vi "DiffVIs.vi"(6 "Title Prefix In":string, 8 "error in":errorcluster, 9 "Picture Save Location":path, 10 "VI Path 2":path, 11 "VI Path 1":path) -> (0 "error out":errorcluster, 2 "diff file":path)   [LabVIEW 2015]
uses:
  Utilities/Arguments.ctl
  Screenshots/VI Screenshots.ctl
  Screenshots/Screenshot Info.ctl
  Screenshots/Screenshot Type.ctl
  Utilities/FilePaths.ctl
  Utilities/VIDiff_Utilities.lvlib
  Screenshots/VIDiff_Screenshots.lvlib
panel:
  out "Description":string
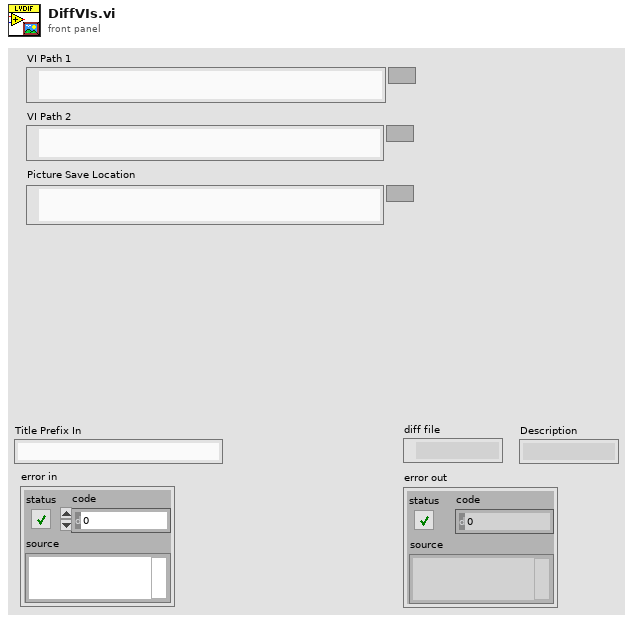
[diagram p1: front panel]
types:
  T1 = typedef "VIDiff_Screenshots.lvlib/Screenshot Type.ctl" = enum16{"Unknown", "Front Panel", "Connector Pane", "Block Diagram", "VI Hierarchy"}
  T2 = typedef "VIDiff_Screenshots.lvlib/VI Screenshots.ctl" = cluster{"Front Panel Screenshots":T3[], "Block Diagram Screenshots":T3[], "Connector Pane Screenshots":T3[], "VI Hierarchy Screenshots":T3[], "Unknown Screenshots":T3[], "vi reference":refnum<vi>, "File Paths":cluster{"File Path":path, "Container Path":path}}
  T3 = typedef "VIDiff_Screenshots.lvlib/Screenshot Info.ctl" = cluster{"Screenshot Path":path, "Screenshot Type":T1, "VI Paths":T4}
  T4 = typedef "VIDiff_Utilities.lvlib/FilePaths.ctl" = cluster{"File Path":path, "Container Path":path}
  T5 = typedef "VIDiff_Utilities.lvlib/Arguments.ctl" = cluster{"VI 1 Path":path, "VI 2 Path":path, "Picture Save Location":path, "Screenshot Title":string}
  T6 = typedef "VIDiff_Utilities.lvlib/Output Folders.ctl" = cluster{"combined":path, "vi1shots":path, "vi2shots":path, "Picture Save Location":path}
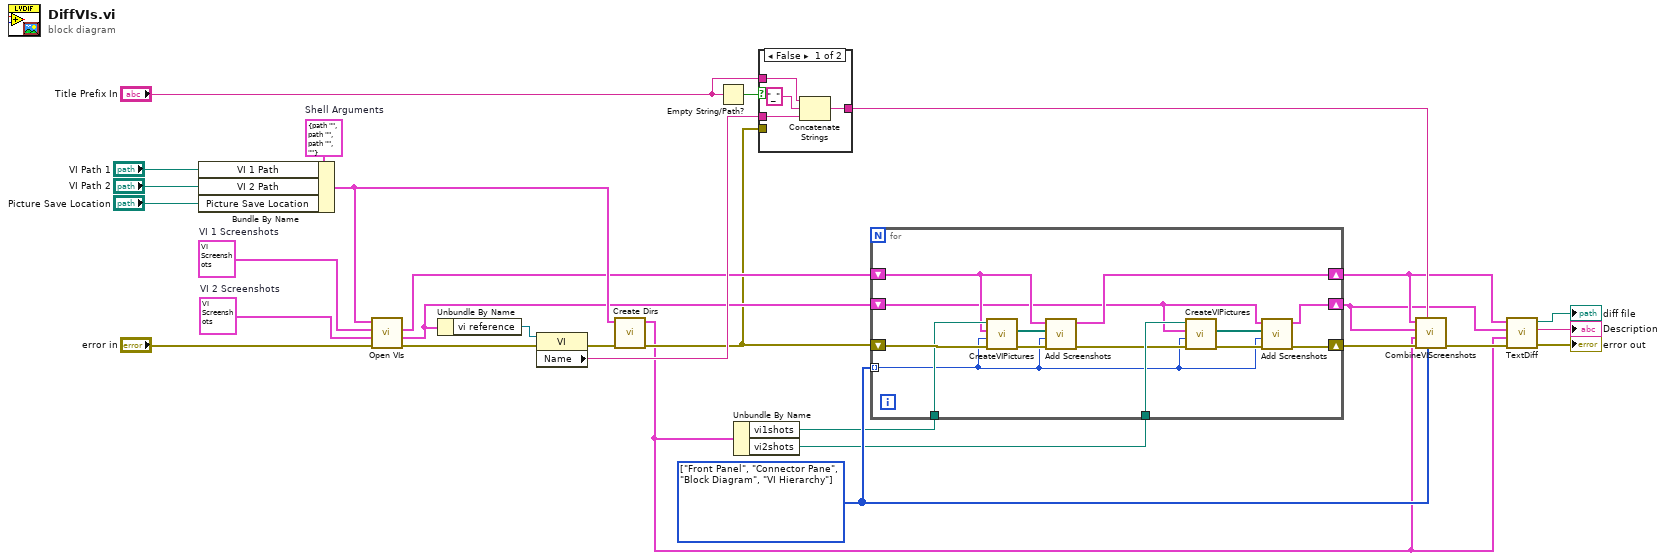
[diagram p0: block diagram]
diagram:
  w17 = T1[] [enum."Front Panel", enum."Connector Pane", enum."Block Diagram", enum."VI Hierarchy"] items=["Unknown", "Front Panel", "Connector Pane", "Block Diagram", "VI Hierarchy"]
  w6 = T2 {"Front Panel Screenshots"=[], "Block Diagram Screenshots"=[], "Connector Pane Screenshots"=[], "VI Hierarchy Screenshots"=[], "Unknown Screenshots"=[], "vi reference"=refnum, "File Paths"={"File Path"=path "", "Container Path"=path ""}}  # VI 2 Screenshots
  w20 = T2 {"Front Panel Screenshots"=[], "Block Diagram Screenshots"=[], "Connector Pane Screenshots"=[], "VI Hierarchy Screenshots"=[], "Unknown Screenshots"=[], "vi reference"=refnum, "File Paths"={"File Path"=path "", "Container Path"=path ""}}  # VI 1 Screenshots
  w29 = T5 {"VI 1 Path"=path "", "VI 2 Path"=path "", "Picture Save Location"=path "", "Screenshot Title"=""}  # Shell Arguments
  n1 = Bundle By Name(cluster=w29, "VI 1 Path"="VI Path 1", "VI 2 Path"="VI Path 2", "Picture Save Location"="Picture Save Location") -> (w21:T5)
  n2 = call "Open VIs.vi"("error in (no error)"="error in", "VI 2 Screenshots 2"=w6, "VI 1 Screenshots"=w20, "Shell Arguments"=w21) -> ("error out"=w10:errorcluster, "VI 2 Screenshots out"=w7:T2, "VI 1 Screenshots out"=w8:T2)  [unwired: 5 in]
  n3 = Unbundle By Name(w7) -> ("vi reference"=w22:refnum<vi>)
  n4 = property class="VI"(reference=w22, error in=w10) -> (error out=w9:errorcluster, "Name"=w13:string)  [unwired: 1 out]
  n5 = call "Create Dirs.vi"("error in (no error)"=w9, "Shell Arguments"=w21) -> ("error out"=w5:errorcluster, "Output Folders"=w2:T6)  [unwired: 8 in]
  n6 = Empty String/Path?(string/path="Title Prefix In") -> (empty?=w19:bool)
  n7 = Unbundle By Name(w2) -> ("vi1shots"=w16:path, "vi2shots"=w15:path)
  n8 = case shown="False" w19 {
    tunnel: w13 -> [w33 w34]
    tunnel: [w32 w34] -> w23
    tunnel: "Title Prefix In" -> [w30 _]
    tunnel: w5 -> [_ _]
    frame False {
      n9 = Concatenate Strings(w30, "_" ("string"), w33) -> (w32:string)
    }
    frame True {
    }
  }
  n10 = for {
    tunnel: w17 -> [w35] mode=indexing
    shift-right: [w43] -> w18
    shift-left: w5 -> [w48]
    tunnel: w16 -> [w47]
    tunnel: w15 -> [w46]
    shift-right: [w42] -> w4
    shift-left: w8 -> [w40]
    shift-right: [w41] -> w3
    shift-left: w7 -> [w39]
    n11 = call "CreateVIPictures.vi"("error in (no error)"=w48, "Capture Target"=w35, "VI 1 Screenshots"=w40, "Picture Save Location"=w47) -> ("error out"=w38:errorcluster, "Screenshot Files"=w45:path[])  [unwired: 6 in]
    n12 = call "Add Screenshots.vi"("error in (no error)"=w38, "Screenshot Type"=w35, "Screenshot Paths"=w45, "VI Screenshots In"=w40) -> ("error out"=w37:errorcluster, "VI Screenshots Out"=w42:T2)  [unwired: 6 in]
    n13 = call "CreateVIPictures.vi"("error in (no error)"=w37, "Capture Target"=w35, "VI 1 Screenshots"=w39, "Picture Save Location"=w46) -> ("error out"=w36:errorcluster, "Screenshot Files"=w44:path[])  [unwired: 6 in]
    n14 = call "Add Screenshots.vi"("error in (no error)"=w36, "Screenshot Type"=w35, "Screenshot Paths"=w44, "VI Screenshots In"=w39) -> ("error out"=w43:errorcluster, "VI Screenshots Out"=w41:T2)  [unwired: 6 in]
  }
  n15 = call "CombineVIScreenshots.vi"("Image Types"=w17, "Name"=w23, "error in (no error)"=w18, "Output Folders"=w2, "VI 2 Screenshots in"=w3, "VI 1 Screenshots in"=w4) -> ("error out"=w11:errorcluster)  [unwired: 5 in]
  n16 = call "TextDiff.vi"("error in (no error)"=w11, "Output Folders"=w2, "VI 2 Screenshots in"=w3, "VI 1 Screenshots in"=w4) -> ("error out"=→"error out":errorcluster, "Description"=→"Description":string, "appended path"=→"diff file":path)  [unwired: 5 in]
